vi "controlAmplitude.vi"(7 "Set":bool, 8 "error in":errorcluster, 9 "amplitude [V]":dbl, 10 "axis in":u8, 11 "connection ID":refnum<k5>) -> (0 "error out":errorcluster, 1 "amplitude [V] out":dbl, 2 "axis out":i32, 3 "connection ID":refnum<k5>)   [LabVIEW 2015, in "AMC_VIs.lvlib"]
doc: "This function retrieves or sets the amplitude of the actuator signal of the selected axis."
uses:
  AMC_VIs.lvlib
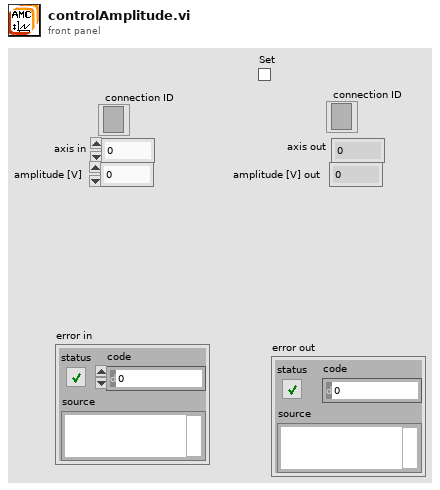
[diagram p1: front panel]
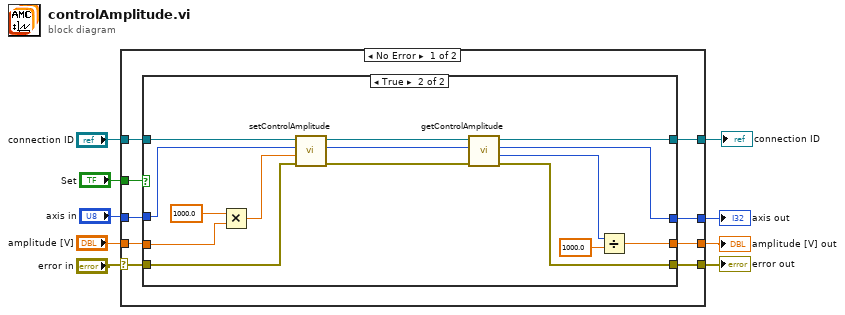
[diagram p0: block diagram]
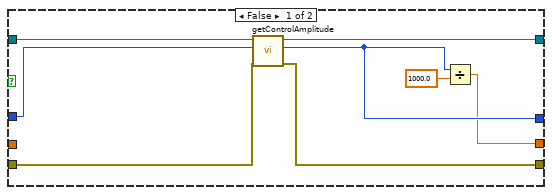
[diagram p2: hidden frame]
diagram:
  n1 = case shown="No Error" "error in" {
    selector: "error in" -> [w12 w45]
    tunnel: "axis in" -> [w18 w42]
    tunnel: [w16 w45] -> w8
    tunnel: "amplitude [V]" -> [w14 w43]
    tunnel: [w11 w43] -> w3
    tunnel: "Set" -> [w13 _]
    tunnel: [w15 w44] -> w6
    tunnel: "connection ID" -> [w17 w44]
    tunnel: [w10 w42] -> w1
    frame No Error {
      n2 = case shown="True" w13 {
        tunnel: [w25 w34] -> w15
        tunnel: w17 -> [w26 w41]
        tunnel: w18 -> [w23 w39]
        tunnel: [w24 w31] -> w16
        tunnel: w14 -> [_ w38]
        tunnel: w12 -> [w22 w40]
        tunnel: [w19 w28] -> w11
        tunnel: [w20 w33] -> w10
        frame False {
          n3 = call "getControlAmplitude.vi"("error in"=w22, "axis"=w23, "connection ID"=w26) -> ("error out"=w24:errorcluster, "axis_out"=w20:i32, "connection ID"=w25:refnum<k5>)  [unwired: 5 in, 1 out]
          n4 = Divide(x=w20, y=1000.0 ("x")) -> (x/y=w19:dbl)
        }
        frame True {
          n5 = Multiply(x=1000.0, y=w38) -> (x*y=w29:dbl)
          n6 = call "setControlAmplitude.vi"("error in"=w40, "amplitude"=w29, "axis"=w39, "connection ID"=w41) -> ("error out"=w32:errorcluster, "axis_out"=w35:i32, "connection ID"=w36:refnum<k5>)  [unwired: 5 in]
          n7 = call "getControlAmplitude.vi"("error in"=w32, "axis"=w35, "connection ID"=w36) -> ("error out"=w31:errorcluster, "amplitude"=w30:i32, "axis_out"=w33:i32, "connection ID"=w34:refnum<k5>)  [unwired: 5 in]
          n8 = Divide(x=w30, y=1000.0 ("x")) -> (x/y=w28:dbl)
        }
      }
    }
    frame Error {
    }
  }
  "error out" <- w8
  "axis out" <- w1
  "amplitude [V] out" <- w3
  "connection ID" <- w6
